vi "Read (Single Point).vi"(8 "error in (no error)":errorcluster, 11 "VISA resource name":refnum<visa-resource-name>) -> (0 "error out":errorcluster, 2 "Measurement":dbl format="%#_8f", 3 "VISA resource name out":refnum<visa-resource-name>)   [LabVIEW 2015, in "Keysight U1252.lvlib"]
doc: "Reads and returns a single measurement from the instrument."
uses:
  <instrlib>/Keysight U1252/Keysight U1252.lvlib
panel:
  out "read buffer":string
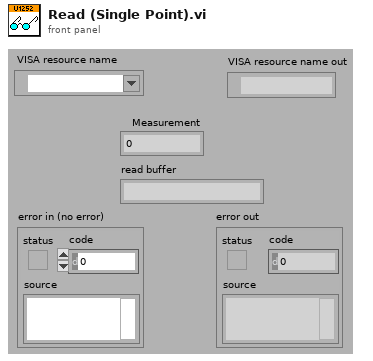
[diagram p1: front panel]
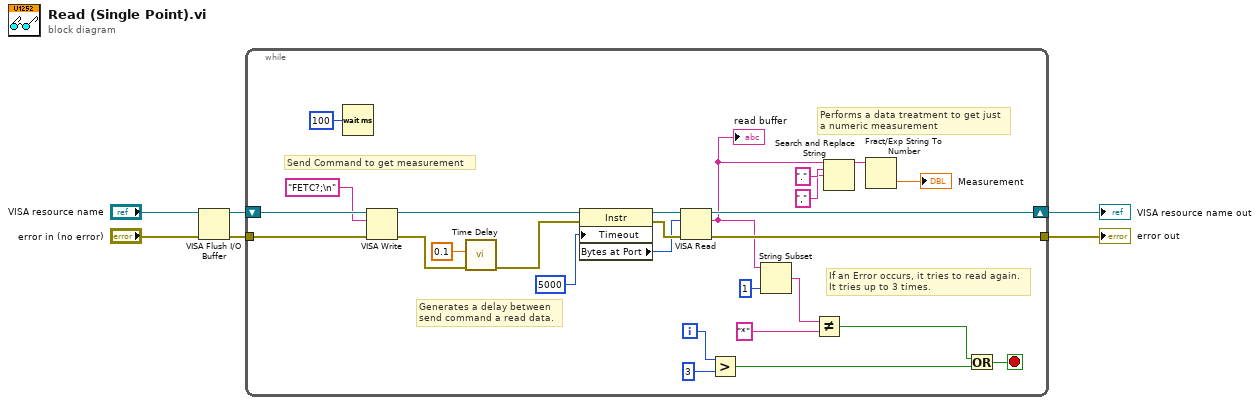
[diagram p0: block diagram]
diagram:
  n1 = VISA Flush I/O Buffer(VISA resource name="VISA resource name", error in (no error)="error in (no error)") -> (VISA resource name out=w3:refnum<visa-resource-name>, error out=w4:errorcluster)  [unwired: 1 in]
  n2 = while {
    shift-right: [w32] -> w5
    shift-left: w3 -> [w33]
    tunnel: w4 -> [w21]
    tunnel: [w18] -> w6
    i -> [w23]
    stop <- w8 stop-if-true
    # "If an Error occurs, it tries to read again.\nIt tries up to 3 times."
    # "Generates a delay between\nsend command a read data."
    # "Performs a data treatment to get just\na numeric measurement"
    # "Send Command to get measurement"
    n3 = Wait (ms)(milliseconds to wait=u32 100) -> ()  [unwired: 1 out]
    n4 = VISA Write(VISA resource name=w33, write buffer="FETC?;\n", error in (no error)=w21) -> (VISA resource name out=w27:refnum<visa-resource-name>, error out=w11:errorcluster)  [unwired: 1 out]
    n5 = call "Time Delay"("error in (no error)"=w11, "Delay Time (s)"=0.1) -> ("error out"=w10:errorcluster)  [unwired: 9 in]
    n6 = property class="Instr"(reference=w27, error in=w10, "Timeout"=u32 5000 ("General Settings:Timeout Value")) -> (reference out=w25:refnum<visa-resource-name>, error out=w24:errorcluster, "Bytes at Port"=w13:u32)
    n7 = VISA Read(VISA resource name=w25, byte count=w13, error in (no error)=w24) -> (VISA resource name out=w32:refnum<visa-resource-name>, read buffer=w16:string, error out=w18:errorcluster)  [unwired: 1 out]
    "read buffer" <- w16
    n8 = Greater?(x=w23, y=3) -> (0:w7:bool)
    n9 = String Subset(string=w16, length (rest)=1 ("length (rest)")) -> (substring=w14:string)  [unwired: 1 in]
    n10 = Not Equal?(x=w14, y="*") -> (x != y?=w9:bool)
    n11 = Search and Replace String(input string=w16, search string=".", replace string="," ("replace string (\"\")")) -> (result string=w28:string)  [unwired: 5 in, 3 out]
    n12 = Fract/Exp String To Number(string=w28) -> (number=→"Measurement":dbl)  [unwired: 3 in, 1 out]
    n13 = Or(x=w9, y=w7) -> (x .or. y?=w8:bool)
  }
  "error out" <- w6
  "VISA resource name out" <- w5
